vi "example_control_access_mode_speed_comparison.vi"() -> ()   [LabVIEW 2015]
doc: "Based on: http://forums.ni.com/ni/board/message?board.id=170&message.id=153531&jump=true"
uses:
  polys/poly_now_high_resolution.vi
  <vilib>/Utility/High Resolution Relative Seconds.vi
  misc_tools/polys/poly_lock_fp_updates_lock_self.vi
  misc_tools/polys/poly_lock_fp_updates_unlock_self.vi
panel:
  out "Method\nName by ref":dbl
  in  "relative?":bool
  out "Property Node\nWrite FP lock":dbl
  out "Property Node\nRead FP lock":dbl
  out "Method":dbl
  out "Property Node\nWrite (Sig.)":dbl
  out "Local Variable\nBoth":dbl
  out "Local Variable\nWrite":dbl
  out "Property Node\nWrite":dbl
  out "Property Node\nRead":dbl
  in  "iterations":i32=10000
  out "Direct\nno loop":dbl
  out "times / multiple of 'direct in loop'":dbl[](array[numeric]) caption="time per iteration / multiple of 'direct in loop'" format="%-.1p"
  out "Direct\nin loop":dbl
  out "Local Variable\nRead":dbl
  # "Baseline"
  # "Much faster\nbecause writes only once"
  # "Little overhead"
  # "Very bad"
  # "Not too bad"
  # "Very bad"
  # "Faster than w\\out\nlock but still bad"
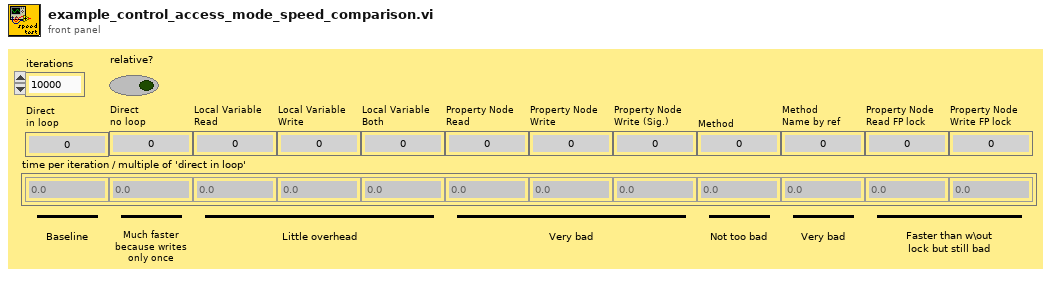
[diagram p1: front panel]
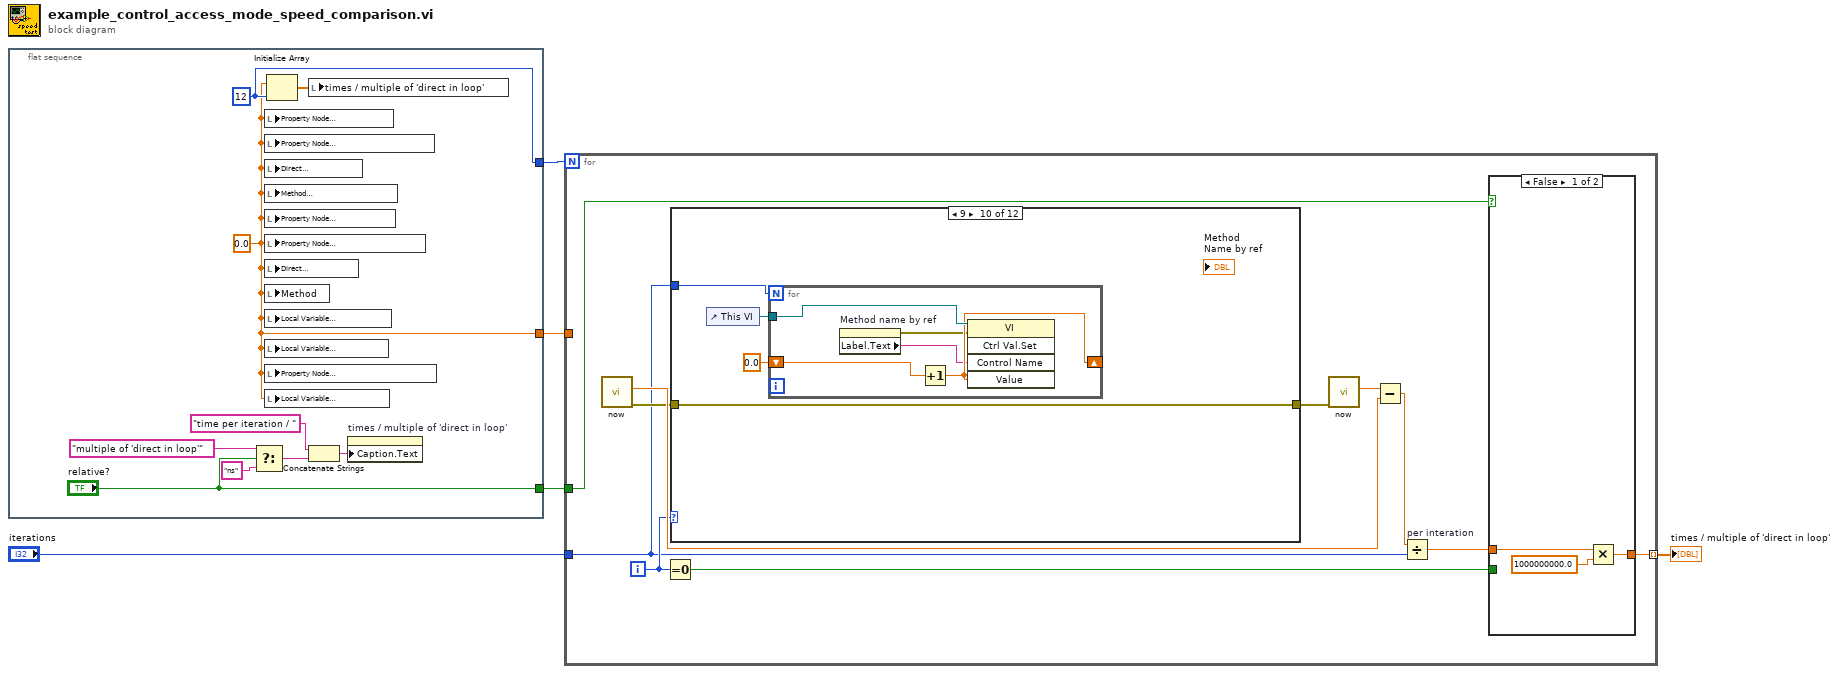
[diagram p0: block diagram]
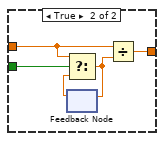
[diagram p2: hidden frame]
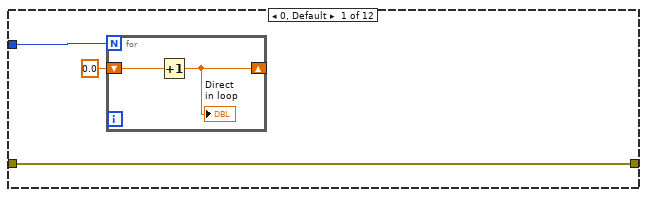
[diagram p3: hidden frame]
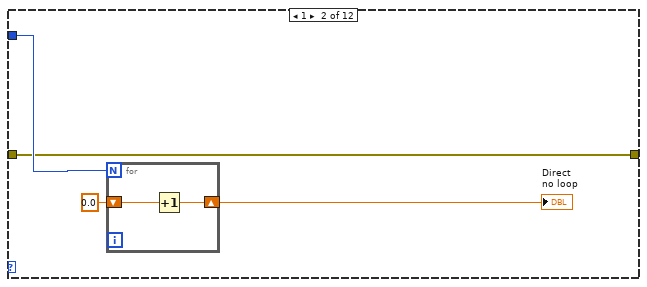
[diagram p4: hidden frame]
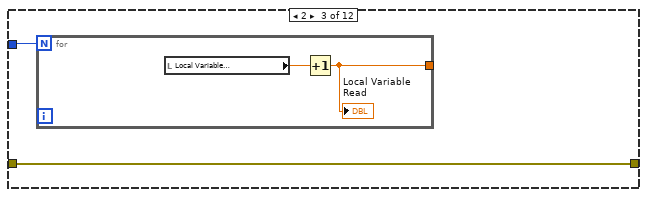
[diagram p5: hidden frame]
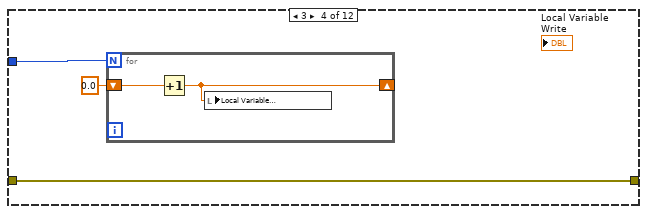
[diagram p6: hidden frame]
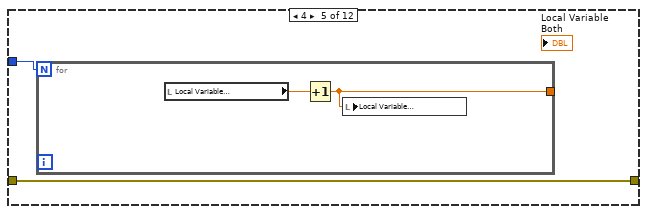
[diagram p7: hidden frame]
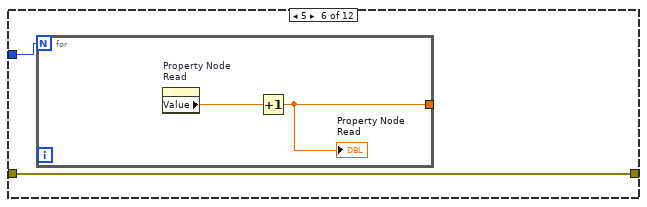
[diagram p8: hidden frame]
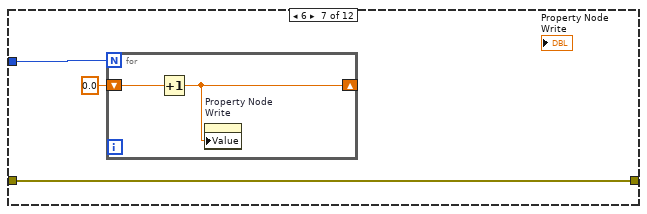
[diagram p9: hidden frame]
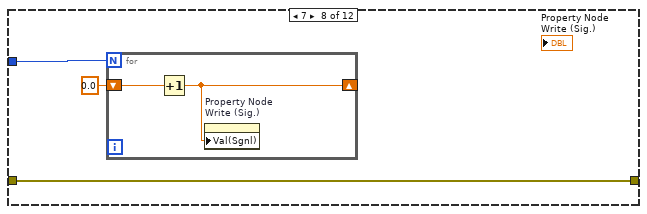
[diagram p10: hidden frame]
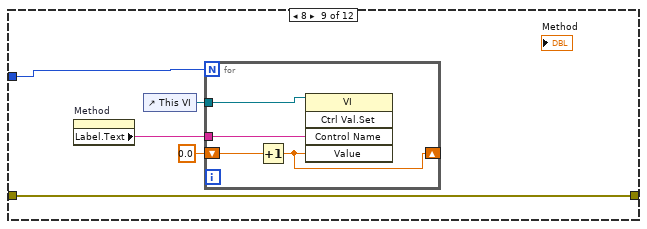
[diagram p11: hidden frame]
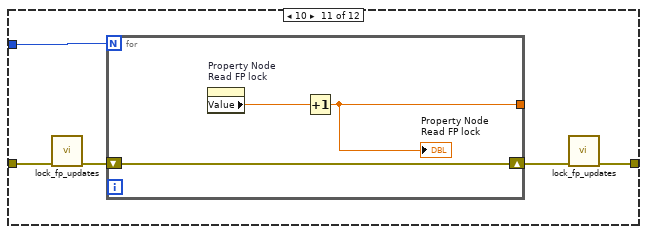
[diagram p12: hidden frame]
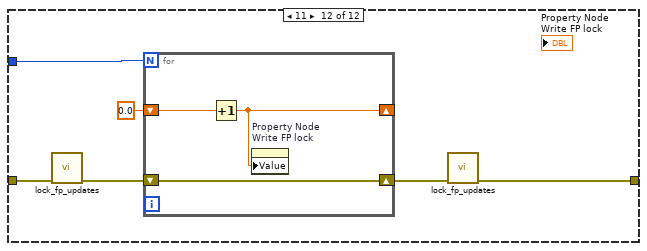
[diagram p13: hidden frame]
diagram:
  n1 = flat-sequence {
    tunnel: [w6] -> w3
    tunnel: [w13] -> w2
    tunnel: ["relative?"] -> w1
    frame #0 {
      w13 = 12
      w6 = 0.0 ("Local Variable")
      n2 = Select(t="multiple of 'direct in loop'", s="relative?", f="ns") -> (s? t:f=w8:string)
      n3 = local write "Property Node\nRead"(w6) -> ()
      n4 = local write "Property Node\nRead FP lock"(w6) -> ()
      n5 = local write "Direct\nno loop"(w6) -> ()
      n6 = local write "Method\nName by ref"(w6) -> ()
      n7 = local write "Property Node\nWrite"(w6) -> ()
      n8 = local write "Property Node\nWrite (Sig.)"(w6) -> ()
      n9 = local write "Direct\nin loop"(w6) -> ()
      n10 = local write "Method"(w6) -> ()
      n11 = local write "Local Variable\nWrite"(w6) -> ()
      n12 = local write "Local Variable\nBoth"(w6) -> ()
      n13 = local write "Property Node\nWrite FP lock"(w6) -> ()
      n14 = local write "Local Variable\nRead"(w6) -> ()
      n15 = Initialize Array(w6, w13) -> (w14:dbl[])
      n16 = local write "times / multiple of 'direct in loop'"(w14) -> ()
      n17 = Concatenate Strings("time per iteration / ", w8) -> (w7:string)
      n18 = property on="times / multiple of 'direct in loop'" class="Arr (strict)"("Caption.Text"=w7) -> ()  [unwired: 2 in, 2 out]
    }
  }
  n19 = for {
    N: w2 -> [_]
    tunnel: [w19] -> w5 mode=indexing
    tunnel: "iterations" -> [w18]
    tunnel: w3 -> [_]
    tunnel: w1 -> [w15]
    i -> [w21]
    n20 = call-poly "now.vi"() -> ("Error out"=w23:errorcluster, "relative seconds"=w24:dbl)  [unwired: 10 in]
    n21 = Equal To 0?(x=w21) -> (x = 0?=w20:bool)
    n22 = case shown="9" w21 {
      tunnel: w18 -> [w35 w41 w46 w51 w55 w59 w64 w69 w76 w84 w94 w103]
      tunnel: w23 -> [w34 w39 w45 w49 w54 w58 w62 w67 w72 w81 w93 w99]
      tunnel: [w34 w39 w45 w49 w54 w58 w62 w67 w72 w81 w90 w98] -> w22
      frame 0, Default {
        n23 = for {
          N: w35 -> [_]
          shift-right: [w37] -> _
          shift-left: 0.0 -> [w38]
          n24 = Increment(x=w38) -> (x+1=w37:dbl)
          "Direct\nin loop" <- w37
        }
      }
      frame 1 {
        n25 = for {
          N: w41 -> [_]
          shift-right: [w43] -> w40
          shift-left: 0.0 -> [w44]
          n26 = Increment(x=w44) -> (x+1=w43:dbl)
        }
        "Direct\nno loop" <- w40
      }
      frame 2 {
        n27 = for {
          N: w46 -> [_]
          tunnel: [w47] -> _
          n28 = local read "Local Variable\nRead"() -> (w48:dbl)
          n29 = Increment(x=w48) -> (x+1=w47:dbl)
          "Local Variable\nRead" <- w47
        }
      }
      frame 3 {
        n30 = for {
          N: w51 -> [_]
          shift-right: [w52] -> _
          shift-left: 0.0 -> [w53]
          n31 = Increment(x=w53) -> (x+1=w52:dbl)
          n32 = local write "Local Variable\nWrite"(w52) -> ()
        }
      }
      frame 4 {
        n33 = for {
          N: w55 -> [_]
          tunnel: [w56] -> _
          n34 = local read "Local Variable\nBoth"() -> (w57:dbl)
          n35 = Increment(x=w57) -> (x+1=w56:dbl)
          n36 = local write "Local Variable\nBoth"(w56) -> ()
        }
      }
      frame 5 {
        n37 = for {
          N: w59 -> [_]
          tunnel: [w60] -> _
          n38 = property on="Property Node\nRead" class="DigNum (strict)"() -> ("Value"=w61:dbl)  [unwired: 2 in, 2 out]
          n39 = Increment(x=w61) -> (x+1=w60:dbl)
          "Property Node\nRead" <- w60
        }
      }
      frame 6 {
        n40 = for {
          N: w64 -> [_]
          shift-right: [w65] -> _
          shift-left: 0.0 -> [w66]
          n41 = Increment(x=w66) -> (x+1=w65:dbl)
          n42 = property on="Property Node\nWrite" class="DigNum (strict)"("Value"=w65) -> ()  [unwired: 2 in, 2 out]
        }
      }
      frame 7 {
        n43 = for {
          N: w69 -> [_]
          shift-right: [w70] -> _
          shift-left: 0.0 -> [w71]
          n44 = Increment(x=w71) -> (x+1=w70:dbl)
          n45 = property on="Property Node\nWrite (Sig.)" class="DigNum (strict)"("Val(Sgnl)"=w70) -> ()  [unwired: 2 in, 2 out]
        }
      }
      frame 8 {
        n46 = property on="Method" class="DigNum (strict)"() -> ("Label.Text"=w73:string)  [unwired: 2 in, 2 out]
        n47 = control-ref of="This VI"() -> (w74:refnum<vi>)
        n48 = for {
          N: w76 -> [_]
          shift-right: [w77] -> _
          shift-left: 0.0 -> [w80]
          tunnel: w74 -> [w79]
          tunnel: w73 -> [w78]
          n49 = Increment(x=w80) -> (x+1=w77:dbl)
          n50 = invoke class="VI" method="Ctrl Val.Set"(reference=w79, "Control Name"=w78, "Value"=w77) -> ()  [unwired: 2 in, 5 out]
        }
      }
      frame 9 {
        n51 = control-ref of="This VI"() -> (w82:refnum<vi>)
        n52 = for {
          N: w84 -> [_]
          shift-right: [w87] -> _
          shift-left: 0.0 -> [w89]
          tunnel: w82 -> [w88]
          n53 = property on="Method name by ref" class="DigNum (strict)"() -> (error out=w85:errorcluster, "Label.Text"=w86:string)  [unwired: 2 in, 1 out]
          n54 = Increment(x=w89) -> (x+1=w87:dbl)
          n55 = invoke class="VI" method="Ctrl Val.Set"(reference=w88, error in=w85, "Control Name"=w86, "Value"=w87) -> ()  [unwired: 1 in, 5 out]
        }
      }
      frame 10 {
        n56 = call-poly "lock_fp_updates.vi"("error in"=w93) -> ("error out"=w92:errorcluster)  [unwired: 10 in]
        n57 = for {
          N: w94 -> [_]
          tunnel: [w97] -> _
          shift-right: [w96] -> w91
          shift-left: w92 -> [w96]
          n58 = property on="Property Node\nRead FP lock" class="DigNum (strict)"() -> ("Value"=w95:dbl)  [unwired: 2 in, 2 out]
          n59 = Increment(x=w95) -> (x+1=w97:dbl)
          "Property Node\nRead FP lock" <- w97
        }
        n60 = call-poly "lock_fp_updates.vi"("error in"=w91) -> ("error out"=w90:errorcluster)  [unwired: 10 in]
      }
      frame 11 {
        n61 = call-poly "lock_fp_updates.vi"("error in"=w99) -> ("error out"=w101:errorcluster)  [unwired: 10 in]
        n62 = for {
          N: w103 -> [_]
          shift-right: [w105] -> _
          shift-left: 0.0 -> [w106]
          shift-right: [w104] -> w100
          shift-left: w101 -> [w104]
          n63 = Increment(x=w106) -> (x+1=w105:dbl)
          n64 = property on="Property Node\nWrite FP lock" class="DigNum (strict)"("Value"=w105) -> ()  [unwired: 2 in, 2 out]
        }
        n65 = call-poly "lock_fp_updates.vi"("error in"=w100) -> ("error out"=w98:errorcluster)  [unwired: 10 in]
      }
    }
    n66 = call-poly "now.vi"("Error in"=w22) -> ("relative seconds"=w25:dbl)  [unwired: 9 in, 1 out]
    n67 = Subtract(x=w25, y=w24) -> (x-y=w16:dbl)
    n68 = Divide "per interation"(x=w16, y=w18) -> (x/y=w17:dbl)
    n69 = case shown="False" w15 {
      tunnel: w20 -> [_ w33]
      tunnel: [w27 w30] -> w19
      tunnel: w17 -> [w28 w29]
      frame False {
        n70 = Multiply(x=w28, y=1000000000.0) -> (x*y=w27:dbl)
      }
      frame True {
        n71 = feedback #1() -> (w32:dbl)  [unwired: 1 in]
        n72 = Select(t=w29, s=w33, f=w32) -> (s? t:f=w31:dbl)
        n73 = feedback-in #1(w31) -> ()
        n74 = Divide(x=w29, y=w31) -> (x/y=w30:dbl)
      }
    }
  }
  "times / multiple of 'direct in loop'" <- w5
